vi "GA Pt Remain.vi"(8 "error in (no error)":errorcluster caption="错误输入（无错误）", 9 "nCount":i16, 10 "pRemainSpace":i32, 11 "nAxisNum":i16) -> (0 "error out":errorcluster caption="错误输出", 2 "pRemainSpace out":i32, 3 "function return":i32)   [LabVIEW 2015, in "GAS.lvlib"]
doc: "extern \"C\" __declspec(dllimport) int GA_PtRemain(short nAxisNum,long *pRemainSpace,short nCount);"
uses:
  <userlib>/BP_GAS/GAS.lvlib
  <userlib>/BP_GAS/GAS.dll
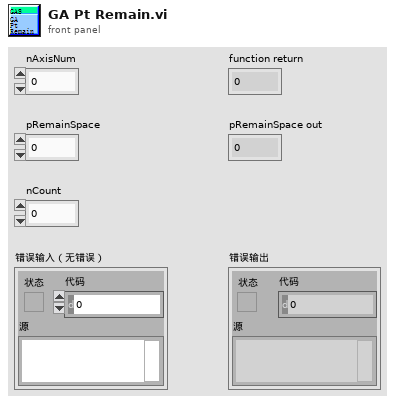
[diagram p1: front panel]
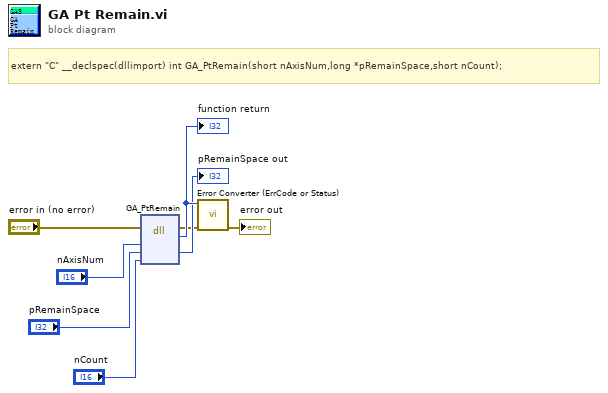
[diagram p0: block diagram]
diagram:
  # "extern \"C\" __declspec(dllimport) int GA_PtRemain(short nAxisNum,long *pRemainSpace,short nCount);"
  n1 = dll-call lib="E:/Program Files (x86)/National Instruments/LabVIEW 2015/user.lib/BP_GAS/GAS.*" fn="GA_PtRemain"(error in="error in (no error)", "nAxisNum"="nAxisNum", "pRemainSpace"="pRemainSpace", "nCount"="nCount") -> (error out=w2:errorcluster, w8:i32, "pRemainSpace"=→"pRemainSpace out":i32)  [unwired: 4 in, 1 out]
  "function return" <- w8
  n2 = call "Error Converter (ErrCode or Status).vi"("error in (no error)"=w2, "error code"=w8) -> ("error out"=→"error out":errorcluster)  [unwired: 9 in]
